vi "GetTorque.vi"(9 "HighSpeedEServer":refnum<k24>, 11 "error in (no error)":errorcluster) -> (1 "Axes":i32[](array[numeric]), 3 "error out":errorcluster)   [LabVIEW 2019, in "UnderAutomation.Yaskawa.lvlib"]
uses:
  UnderAutomation.Yaskawa.lvlib
  C:/Users/fg/Documents/Yaskawa.vi/LabVIEW_2024/UnderAutomation.Yaskawa/lib/UnderAutomation.Yaskawa.dll
  LabVIEW_2024/UnderAutomation.Yaskawa/lib/UnderAutomation.Yaskawa.dll
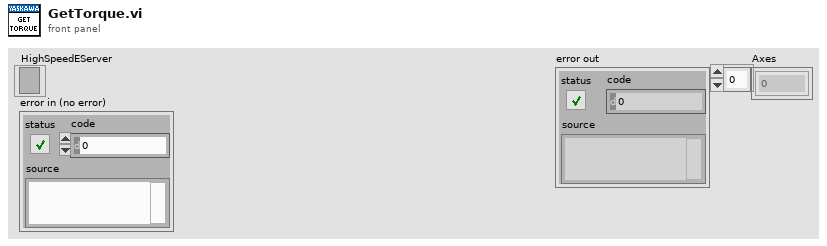
[diagram p1: front panel]
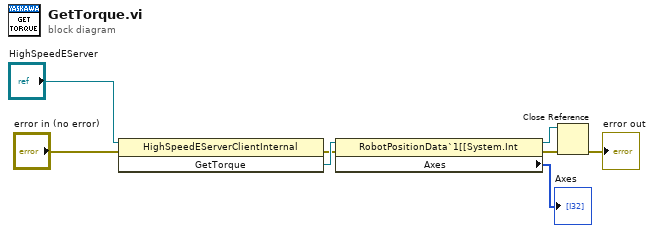
[diagram p0: block diagram]
diagram:
  n1 = invoke class="HighSpeedEServerClientInternal" method="GetTorque"(reference="HighSpeedEServer", error in="error in (no error)") -> (error out=w5:errorcluster, "GetTorque"=w6:refnum<k24>)  [unwired: 1 in, 1 out]
  n2 = property class="RobotPositionData`1[[System.Int"(reference=w6, error in=w5) -> (reference out=w1:refnum<k24>, error out=w3:errorcluster, "Axes"=→"Axes":i32[])
  n3 = Close Reference(reference=w1, error in (no error)=w3) -> (error out=→"error out":errorcluster)
